vi "Get State.vi"(8 "error in (no error)":errorcluster, 11 "Tektronix Driver in":refnum<class "Tektronix 4000 Driver.lvclass">) -> (0 "error out":errorcluster, 1 "Data ready":bool, 2 "Armed":bool, 3 "Tektronix Driver out":refnum<class "Tektronix 4000 Driver.lvclass">, 4 "Availiable Samples":u32, 5 "Finished":bool)   [LabVIEW 2020, in "Tektronix 4000 Driver.lvclass"]
uses:
  Tektronix 4000 Driver.lvclass
  C:/GitHub/NHMFL_Core/Libraries/Instruments/Tektronix/Tektronix Driver/Tektronix Driver.lvclass
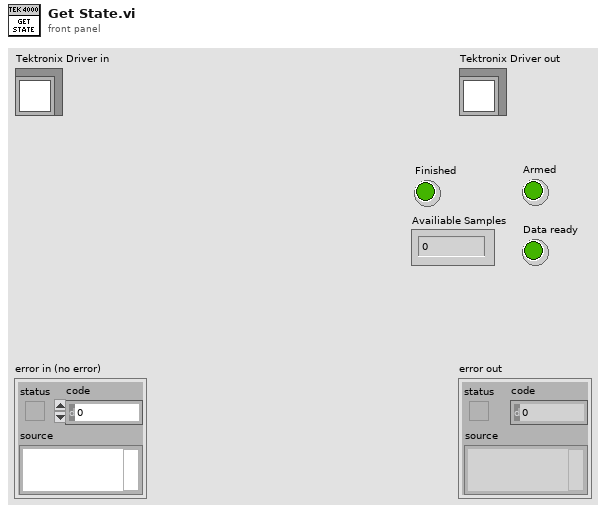
[diagram p1: front panel]
types:
  T1 = typedef "Tektronix Configuration.ctl" = cluster{"Channel":i32, "Number of averages":i32, "Input impedace":enum16{"1 M Ohm", "50 Ohm"}, "Vertical coupling":enum16{"AC", "DC", "Ground"}}
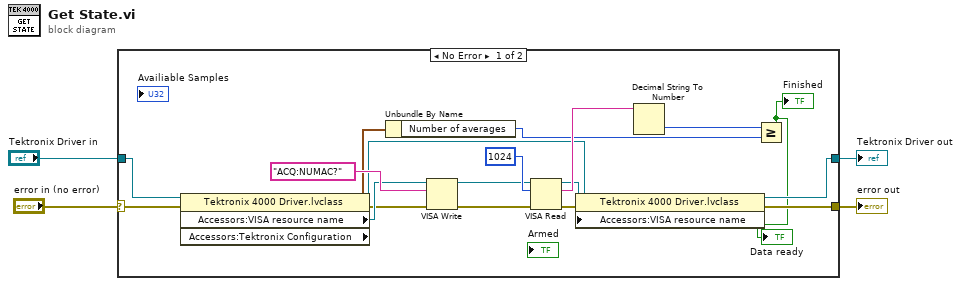
[diagram p0: block diagram]
diagram:
  n1 = case shown="No Error" "error in (no error)" {
    selector: "error in (no error)" -> [w22 w24]
    tunnel: [w9 w24] -> w3
    tunnel: [w7 w23] -> w1
    tunnel: "Tektronix Driver in" -> [w16 w23]
    frame No Error {
      n2 = property class="Tektronix 4000 Driver.lvclass"(reference=w16, error in=w22) -> (reference out=w8:refnum<class "Tektronix 4000 Driver.lvclass">, error out=w13:errorcluster, "Accessors:VISA resource name"=w15:refnum<visa-resource-name>, "Accessors:Tektronix Configuration"=w14:T1)
      n3 = Unbundle By Name(w14) -> ("Number of averages"=w11:i32)
      n4 = VISA Write(VISA resource name=w15, write buffer="ACQ:NUMAC?", error in (no error)=w13) -> (VISA resource name out=w20:refnum<visa-resource-name>, error out=w18:errorcluster)  [unwired: 1 out]
      n5 = VISA Read(VISA resource name=w20, byte count=u32 1024, error in (no error)=w18) -> (VISA resource name out=w6:refnum<visa-resource-name>, read buffer=w17:string, error out=w10:errorcluster)  [unwired: 1 out]
      n6 = property class="Tektronix 4000 Driver.lvclass"(reference=w8, error in=w10, "Accessors:VISA resource name"=w6) -> (reference out=w7:refnum<class "Tektronix 4000 Driver.lvclass">, error out=w9:errorcluster)
      n7 = Decimal String To Number(string=w17) -> (number=w12:i32)  [unwired: 2 in, 1 out]
      n8 = Greater Or Equal?(x=w12, y=w11) -> (x >= y?=→"Finished" →"Data ready":bool)
    }
    frame Error {
    }
  }
  "error out" <- w3
  "Tektronix Driver out" <- w1
